vi "set MFC3 changes.vi"(7 "init":bool, 8 "Fehler (Eingang, kein Fehler)":errorcluster, 9 "Changes":T1, 11 "TestKonfig (Eingang)":T3 {"TestKonfig Interferent"."Gasflasche MFC3" items=["----"=10000, "IAG NH3 3000"=0, "IAG NH3 200"=1, "IAG NH3 2000"=2, "IAG MG"=3, "IAG O2"=4]; "TestKonfig Interferent"."Gasflasche MFC2" items=["----"=10000, "IAG NH3 3000"=0, "IAG NH3 200"=1, "IAG NH3 2000"=2, "IAG MG"=3, "IAG O2"=4]; "TestKonfig Interferent"."Eingangs Konzentration MFC1" min=0.0; "TestKonfig Interferent"."Ausgangs Konzentration MFC1" min=0.0; "TestKonfig Interferent"."MFC2" items=["MFC 2", "MFC 3", "MFC 4", "MFC 5"]; "TestKonfig Interferent"."MFC3" items=["MFC 2", "MFC 3", "MFC 4", "MFC 5"]; "TestKonfig Interferent"."Ausgangs Konzentration MFC3" min=0.0; "TestKonfig Interferent"."Eingangs Konzentration MFC3" min=0.0; "TestKonfig Interferent"."Ausgangs Konzentration MFC2" min=0.0; "TestKonfig Interferent"."Eingangs Konzentration MFC2" min=0.0; "TestKonfig H2O"."HovaCAL Temperature" format="%.2f"; "TestKonfig H2O"."HovaCAL Flow Input Cluster"."HovaCAL Flow Input Cluster" format="%.2f"; "TestKonfig H2O"."Eingangs Konzentration:" min=0.0; "TestKonfig H2O"."zusätzliche Zeitdauer Erster Punkt" min=30 step=1 format="%#_5g"; "TestKonfig H2O"."Zeitdauer Stufen" format="%#_5g"; "TestKonfig H2O"."Max Fehler" format="%#_5g"; "TestKonfig H2O"."Anzahl Stufen" format="%#_5g"; "TestKonfig H2O"."Modus" items=["Messen", "CG zu Entnahmestelle"]}) -> (0 "Fehler (Ausgang)":errorcluster, 1 "Changes  out":T1, 2 "Komponenten Name":T2, 3 "TestKonfig (Ausgang)":T3 {"TestKonfig Interferent"."Gasflasche MFC3" items=["----"=10000, "IAG NH3 3000"=0, "IAG NH3 200"=1, "IAG NH3 2000"=2, "IAG MG"=3, "IAG O2"=4]; "TestKonfig Interferent"."Gasflasche MFC2" items=["----"=10000, "IAG NH3 3000"=0, "IAG NH3 200"=1, "IAG NH3 2000"=2, "IAG MG"=3, "IAG O2"=4]; "TestKonfig Interferent"."Eingangs Konzentration MFC1" min=0.0; "TestKonfig Interferent"."Ausgangs Konzentration MFC1" min=0.0; "TestKonfig Interferent"."MFC2" items=["MFC 2", "MFC 3", "MFC 4", "MFC 5"]; "TestKonfig Interferent"."MFC3" items=["MFC 2", "MFC 3", "MFC 4", "MFC 5"]; "TestKonfig Interferent"."Ausgangs Konzentration MFC3" min=0.0; "TestKonfig Interferent"."Eingangs Konzentration MFC3" min=0.0; "TestKonfig Interferent"."Ausgangs Konzentration MFC2" min=0.0; "TestKonfig Interferent"."Eingangs Konzentration MFC2" min=0.0; "TestKonfig H2O"."HovaCAL Temperature" format="%.2f"; "TestKonfig H2O"."HovaCAL Flow Input Cluster"."HovaCAL Flow Input Cluster" format="%.2f"; "TestKonfig H2O"."Eingangs Konzentration:" min=0.0; "TestKonfig H2O"."zusätzliche Zeitdauer Erster Punkt" min=30 step=1 format="%#_5g"; "TestKonfig H2O"."Zeitdauer Stufen" format="%#_5g"; "TestKonfig H2O"."Max Fehler" format="%#_5g"; "TestKonfig H2O"."Anzahl Stufen" format="%#_5g"; "TestKonfig H2O"."Modus" items=["Messen", "CG zu Entnahmestelle"]})   [LabVIEW 2020, in "EPA 1065.lvlib" / "HovaCAL Interference verificaton.lvlib"]
uses:
  HovaCAL Interference verificaton.lvlib
  TestKonfig.ctl
  TestKonfig H2O.ctl
  Modus.ctl
  Linearisierung V2/SpanEinstellungen/Einheit.ctl
  Linearisierung V2/Gasteiler/Stufen Tabelle 10 Stufen.ctl
  Linearisierung V2/Gasteiler/HovaCAL_Interface/Controls/Flow Einstellung.ctl
  Linearisierung V2/Gasteiler/HovaCAL_Interface/Controls/Temp Sollwerte Anzeige.ctl
  TestKonfig Interferents.ctl
  MFCAuswahl.ctl
  Seiten/System Einstellungen V2/Gasflasche Auswahl.ctl
  Visualisierungs Elemente/String - Ausgabefeld.ctl
  Konfig changes.ctl
  Aktion Index uebersetzten.ctl
  Linearisierung V2/Gasteiler/Gasteiler.lvlib
  Linearisierung V2/SpanEinstellungen/SpanEinstellungen.lvlib
  Linearisierung V2/Gasteiler/HovaCAL_Interface/Controls/Controls.lvlib
  Seiten/System Einstellungen V2/System Einstellungen V2.lvlib
panel:
  # "sec"
  # "%"
  # "sec"
  # "sec"
  # "%"
  # "sec"
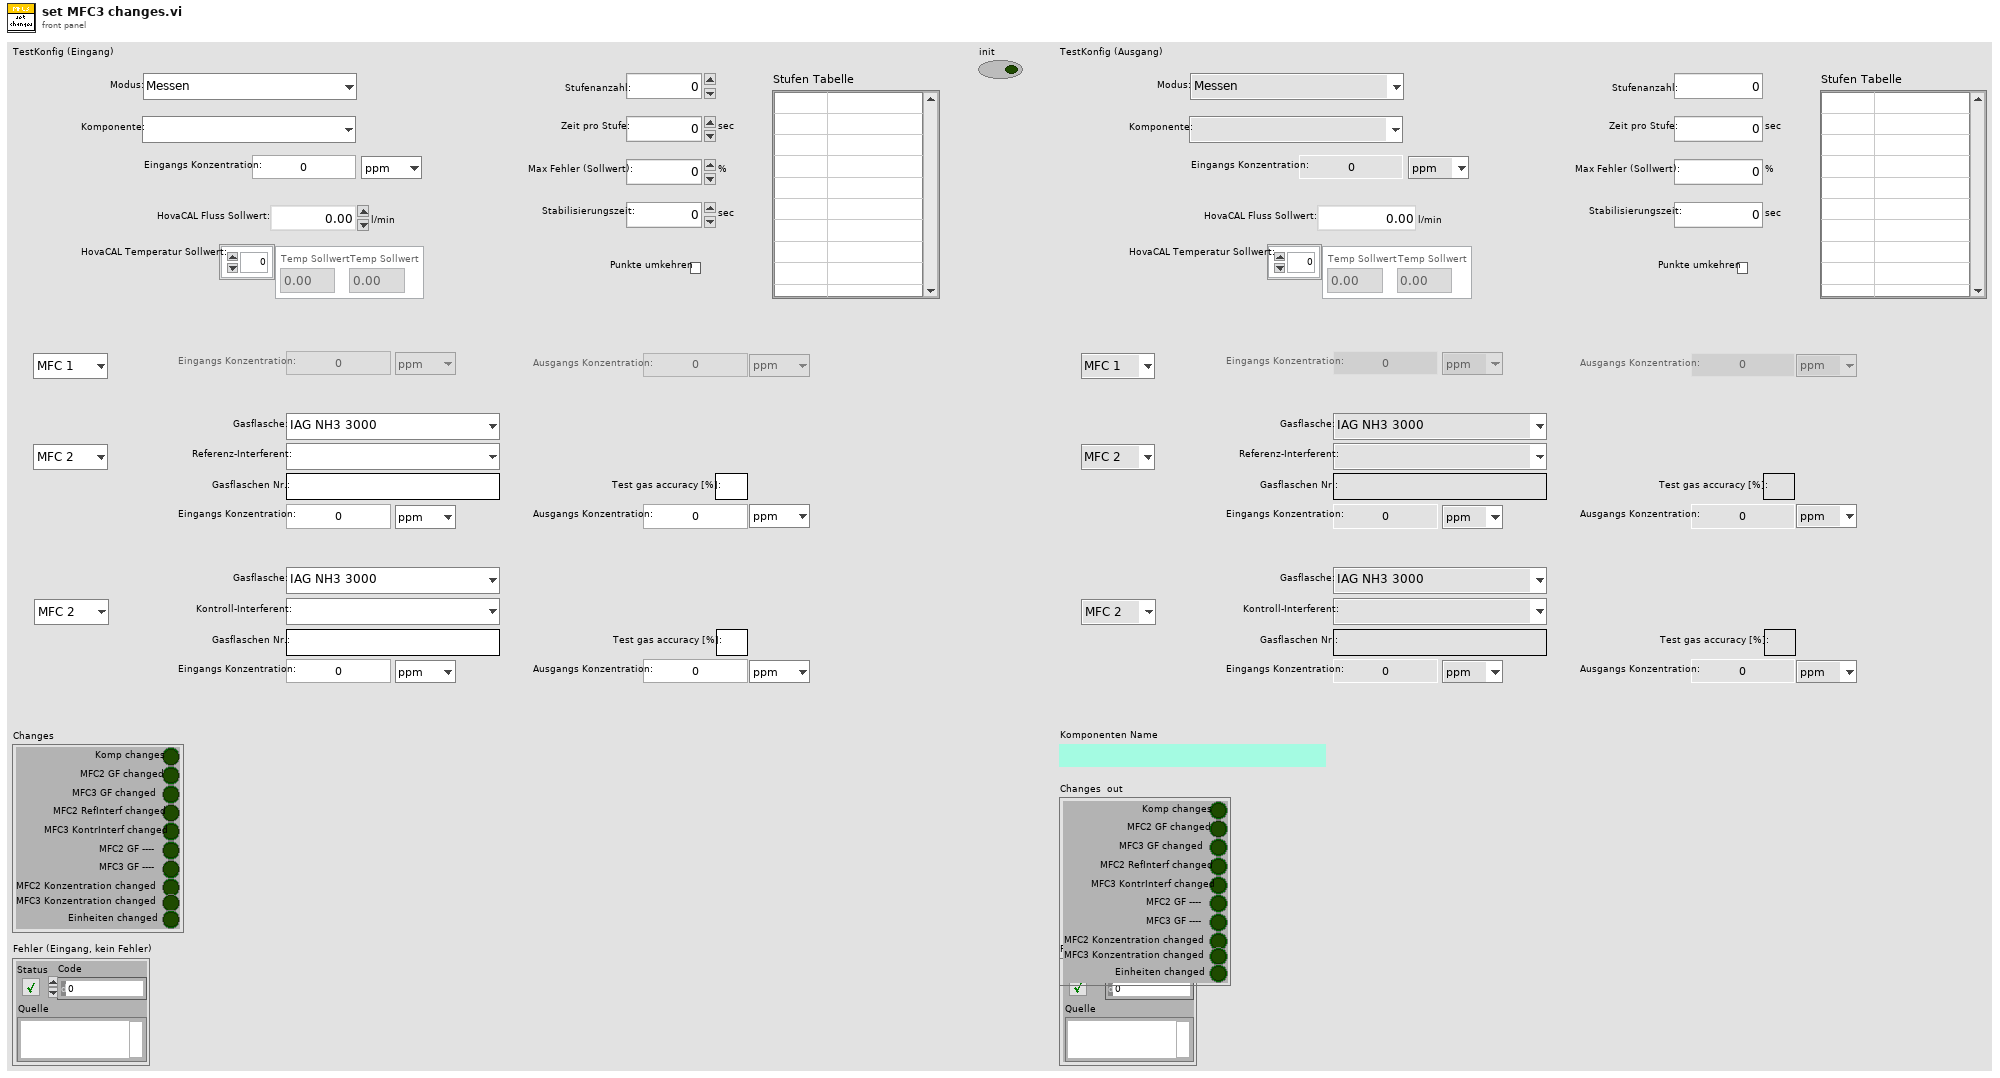
[diagram p1: front panel]
types:
  T1 = typedef "EPA 1065.lvlib/HovaCAL Interference verificaton.lvlib/Konfig changes.ctl" = cluster{"Komp changes":bool, "MFC2 GF changed":bool, "MFC3 GF changed":bool, "MFC2 RefInterf changed":bool, "MFC3 KontrInterf changed":bool, "MFC2 GF ----":bool, "MFC3 GF ----":bool, "MFC2 Konzentration changed":bool, "MFC3 Konzentration changed":bool, "Einheiten changed":bool}
  T2 = typedef "String - Ausgabefeld.ctl" = string
  T3 = typedef "EPA 1065.lvlib/HovaCAL Interference verificaton.lvlib/TestKonfig.ctl" = cluster{"TestKonfig H2O":T4, "TestKonfig Interferent":T10}
  T4 = typedef "EPA 1065.lvlib/HovaCAL Interference verificaton.lvlib/TestKonfig H2O.ctl" = cluster{"Modus":T5, "Komponente:":u16, "Eingangs Konzentration:":dbl, "Einheit":T6, "Anzahl Stufen":sgl, "Zeitdauer Stufen":sgl, "Max Fehler":sgl, "zusätzliche Zeitdauer Erster Punkt":sgl, "Punkte umkehren":bool, "Stufen Tabelle":T7, "HovaCAL Flow Input Cluster":T8, "HovaCAL Temperature":T9}
  T5 = typedef "EPA 1065.lvlib/HovaCAL Interference verificaton.lvlib/Modus.ctl" = u16
  T6 = typedef "Linearisierung v2.lvlib/SpanEinstellungen.lvlib/Einheit.ctl" = enum16{"ppm", "%"}
  T7 = typedef "Linearisierung v2.lvlib/Gasteiler.lvlib/Stufen Tabelle 10 Stufen.ctl" = string[][]
  T8 = typedef "Linearisierung v2.lvlib/Gasteiler.lvlib/HovaCAL_Interface.lvlib/Controls.lvlib/Flow Einstellung.ctl" = cluster{"HovaCAL Flow Input Cluster":dbl}
  T9 = typedef "Linearisierung v2.lvlib/Gasteiler.lvlib/HovaCAL_Interface.lvlib/Controls.lvlib/Temp Sollwerte Anzeige.ctl" = dbl[]
  T10 = typedef "EPA 1065.lvlib/HovaCAL Interference verificaton.lvlib/TestKonfig Interferents.ctl" = cluster{"MFC1":enum16{"MFC 1"}, "Eingangs Konzentration MFC1":dbl, "Einheit MFC1 Eingang":T6, "Ausgangs Konzentration MFC1":dbl, "Einheit MFC1 Ausgang":T6, "MFC2":T11, "Referenz-Interferent:":u16, "Gasflaschen Nr MFC2":string, "Accuracy MFC2":string, "Eingangs Konzentration MFC2":dbl, "Einheit MFC2 Eingang":T6, "Ausgangs Konzentration MFC2":dbl, "Einheit MFC2 Ausgang":T6, "MFC3":T11, "Kontroll-Interferent:":u16, "Gasflaschen Nr MFC3":string, "Accuracy MFC3":string, "Eingangs Konzentration MFC3":dbl, "Einheit MFC3 Eingang":T6, "Ausgangs Konzentration MFC3":dbl, "Einheit MFC3 Ausgang":T6, "Gasflasche MFC2":T12, "Gasflasche MFC3":T12}
  T11 = typedef "EPA 1065.lvlib/HovaCAL Interference verificaton.lvlib/MFCAuswahl.ctl" = u16
  T12 = typedef "System Einstellungen V2.lvlib/Gasflasche Auswahl.ctl" = u16
  T13 = typedef "EPA 1065.lvlib/HovaCAL Interference verificaton.lvlib/Aktion Index uebersetzten.ctl" = enum16{"lesen", "schreiben", "auswerten", "Referenzwert", "KompIndex", "RefInterferIndex", "KontrInterfIndex"}
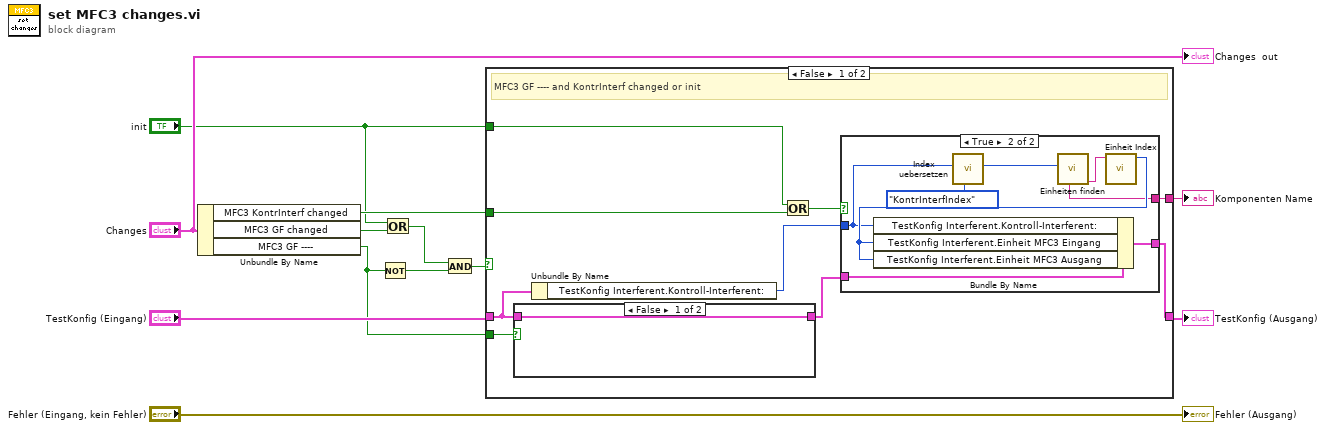
[diagram p0: block diagram]
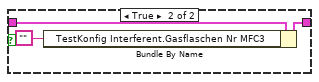
[diagram p2: hidden frame]
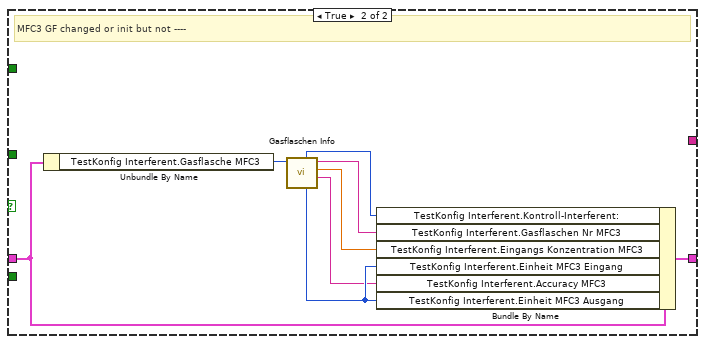
[diagram p4: hidden frame]
diagram:
  n1 = Unbundle By Name("Changes") -> ("MFC3 KontrInterf changed"=w7:bool, "MFC3 GF changed"=w6:bool, "MFC3 GF ----"=w1:bool)
  n2 = Not(x=w1) -> (.not. x?=w3:bool)
  n3 = Or(x="init", y=w6) -> (x .or. y?=w4:bool)
  n4 = And(x=w4, y=w3) -> (x .and. y?=w2:bool)
  n5 = case shown="False" w2 {
    tunnel: "TestKonfig (Eingang)" -> [w18 w36]
    tunnel: [w17 w42] -> w12
    tunnel: "init" -> [w20 _]
    tunnel: [w16 _] -> w10
    tunnel: w7 -> [w15 _]
    tunnel: w1 -> [w13 _]
    frame False {
      # "MFC3 GF ---- and KontrInterf changed or init"
      n6 = case shown="False" w13 {
        tunnel: w18 -> [w22 w25]
        tunnel: [w22 w24] -> w14
        frame False {
        }
        frame True {
          n7 = Bundle By Name(cluster=w25, "TestKonfig Interferent.Gasflaschen Nr MFC3"="") -> (w24:T3)
        }
      }
      n8 = Unbundle By Name(w18) -> ("TestKonfig Interferent.Kontroll-Interferent:"=w19:u16)
      n9 = Or(x=w20, y=w15) -> (x .or. y?=w21:bool)
      n10 = case shown="True" w21 {
        tunnel: w14 -> [w26 w34]
        tunnel: [w26 w33] -> w17
        tunnel: w19 -> [_ w29]
        tunnel: [_ w27] -> w16
        frame False {
        }
        frame True {
          n11 = call "Index uebersetzen.vi"("Aktion"=Aktion_Index_uebersetzten."KontrInterfIndex", "Index relativ:"=w29) -> ("Index absolut"=w28:i32)  [unwired: 4 in, 5 out]
          n12 = call "Einheiten finden.vi"("Komponente"=w28) -> ("Einheit in String"=w32:string, "Komponenten Name"=w27:T2)  [unwired: 6 in, 3 out]
          n13 = call "Einheit Index.vi"("Einheit in String"=w32) -> ("Elementindex"=w31:i32)  [unwired: 10 in]
          n14 = Bundle By Name(cluster=w34, "TestKonfig Interferent.Kontroll-Interferent:"=w29, "TestKonfig Interferent.Einheit MFC3 Eingang"=w31, "TestKonfig Interferent.Einheit MFC3 Ausgang"=w31) -> (w33:T3)
        }
      }
    }
    frame True {
      # "MFC3 GF changed or init but not ----"
      n15 = Unbundle By Name(w36) -> ("TestKonfig Interferent.Gasflasche MFC3"=w35:T12)
      n16 = call "Gasflaschen Info.vi"("Gasflasche MFC2"=w35) -> ("String"=w38:string, "Konzentration IST"=w40:dbl, "Chargennummer"=w41:string, "Einheitindex"=w39:i32, "Component"=w37:i32)  [unwired: 5 in, 1 out]
      n17 = Bundle By Name(cluster=w36, "TestKonfig Interferent.Kontroll-Interferent:"=w37, "TestKonfig Interferent.Gasflaschen Nr MFC3"=w41, "TestKonfig Interferent.Eingangs Konzentration MFC3"=w40, "TestKonfig Interferent.Einheit MFC3 Eingang"=w39, "TestKonfig Interferent.Accuracy MFC3"=w38, "TestKonfig Interferent.Einheit MFC3 Ausgang"=w39) -> (w42:T3)
    }
  }
  "TestKonfig (Ausgang)" <- w12
  "Komponenten Name" <- w10
  "Fehler (Ausgang)" <- "Fehler (Eingang, kein Fehler)"
  "Changes  out" <- "Changes"
